vi "Pre Launch Init.vi"(11 "Nested in":refnum<class "Test Application Controller.lvclass">) -> (0 "error out":errorcluster, 3 "Nested out":refnum<class "Test Application Controller.lvclass">)   [LabVIEW 2017, in "Test Application Controller.lvlib" / "Test Application Controller.lvclass"]
doc: "(<B>Filename</B>: Actor Framework.lvlib:Actor.lvclass:Pre Launch Init.vi)\n\nDefines behavior that occurs after the Launch Nested Actor method is invoked but before the actor's Actor Core method begins running.\n\nBy default, this method does nothing. A descendant class may override it to define behavior."
uses:
  Test Application Controller.lvclass
  Test Application Controller.lvclass/Test Application Controller.ctl
  <vilib>/ActorFramework/Actor/Actor.lvclass
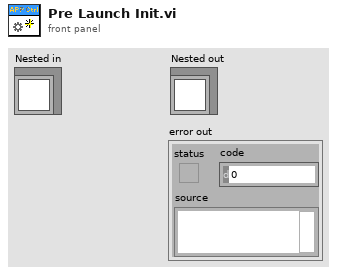
[diagram p1: front panel]
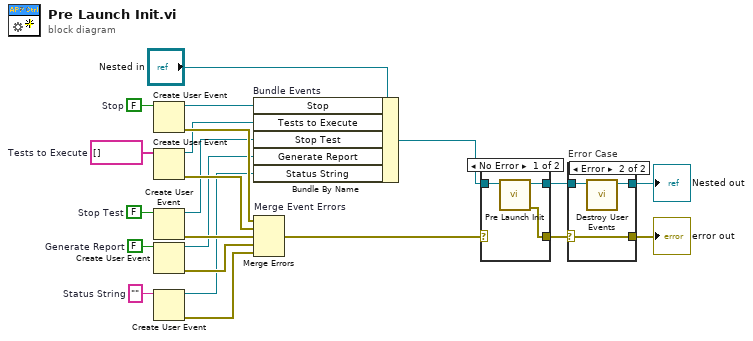
[diagram p0: block diagram]
diagram:
  w3 = ""  # Status String
  w6 = FALSE  # Generate Report
  w9 = FALSE  # Stop Test
  w12 = string[] []  # Tests to Execute
  w21 = FALSE  # Stop
  n1 = Create User Event(user event datatype=w21) -> (user event=w18:refnum<user-event>, error out=w20:errorcluster)  [unwired: 1 in]
  n2 = Create User Event(user event datatype=w12) -> (user event=w11:refnum<user-event>, error out=w10:errorcluster)  [unwired: 1 in]
  n3 = Create User Event(user event datatype=w9) -> (user event=w8:refnum<user-event>, error out=w7:errorcluster)  [unwired: 1 in]
  n4 = Create User Event(user event datatype=w6) -> (user event=w5:refnum<user-event>, error out=w4:errorcluster)  [unwired: 1 in]
  n5 = Create User Event(user event datatype=w3) -> (user event=w2:refnum<user-event>, error out=w1:errorcluster)  [unwired: 1 in]
  n6 = Bundle By Name "Bundle Events"(cluster="Nested in", "Stop"=w18, "Tests to Execute"=w11, "Stop Test"=w8, "Generate Report"=w5, "Status String"=w2) -> (w15:refnum<class "Test Application Controller.lvclass">)
  n7 = Merge Errors "Merge Event Errors"(w20, w10, w7, w4, w1) -> (w14:errorcluster)
  n8 = case shown="No Error" w14 {
    selector: w14 -> [_ w27]
    tunnel: [w25 w26] -> w16
    tunnel: w15 -> [w24 w26]
    tunnel: [w23 w27] -> w13
    frame No Error {
      n9 = call-parent "Pre Launch Init.vi"("Actor in"=w24) -> ("error out"=w23:errorcluster, "Actor out"=w25:refnum<class "Test Application Controller.lvclass">)  [unwired: 9 in]
    }
    frame Error {
    }
  }
  n10 = case "Error Case" shown="Error" w13 {
    selector: w13 -> [w28 w32]
    tunnel: w16 -> [w29 w31]
    tunnel: [w29 w30] -> w19
    tunnel: [w28 w32] -> w17
    frame No Error {
    }
    frame Error {
      n11 = call "Destroy User Events.vi"("UI Template in"=w31) -> ("UI Template out"=w30:refnum<class "Test Application Controller.lvclass">)  [unwired: 10 in]
    }
  }
  "error out" <- w17
  "Nested out" <- w19
